vi "Rename InstrumentStudio Plug-In Data File.vi"(0 "configuration":T1, 5 "Plugin Library Path":path, 11 "error in":errorcluster) -> (4 "IS Plugin Data File Path":path, 15 "error out":errorcluster)   [LabVIEW 2021, in "InstrumentStudio Plug-In Editor.lvlib"]
uses:
  InstrumentStudio Plug-In Editor.lvlib
  controls/Data Holder.ctl
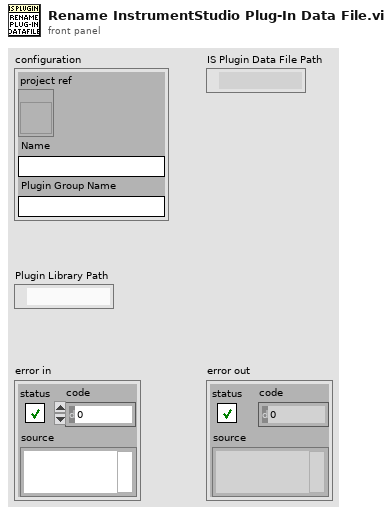
[diagram p1: front panel]
types:
  T1 = typedef "InstrumentStudio Plug-In Editor.lvlib/Data Holder.ctl" = cluster{"project ref":refnum<vi>, "Name":string, "Plugin Group Name":string}
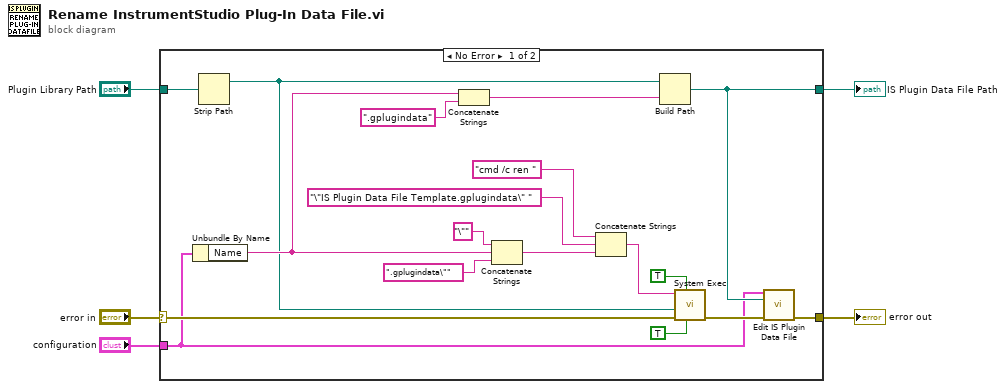
[diagram p0: block diagram]
diagram:
  n1 = case shown="No Error" "error in" {
    selector: "error in" -> [w11 w24]
    tunnel: "Plugin Library Path" -> [w10 _]
    tunnel: [w8 _] -> w3
    tunnel: [w7 w24] -> w2
    tunnel: "configuration" -> [w6 _]
    frame No Error {
      n2 = Unbundle By Name(w6) -> ("Name"=w16:string)
      n3 = Strip Path(path=w10) -> (stripped path=w13:path)  [unwired: 1 out]
      n4 = Concatenate Strings(w16, ".gplugindata" ("string")) -> (w14:string)
      n5 = Concatenate Strings("\"" ("string"), w16, ".gplugindata\"" ("string")) -> (w18:string)
      n6 = Concatenate Strings("cmd /c ren " ("string"), "\"IS Plugin Data File Template.gplugindata\" " ("string"), w18) -> (w21:string)
      n7 = Build Path(base path=w13, name or relative path=w14) -> (appended path=w8:path)
      n8 = call <vilib>:"System Exec.vi"("run minimized? (F)"=TRUE, "wait until completion? (T)"=TRUE, "error in (no error)"=w11, "working directory"=w13, "command line"=w21) -> ("error out"=w9:errorcluster)  [unwired: 3 in, 3 out]
      n9 = call "Edit IS Plugin Data File.vi"("configuration"=w6, "Data File Path"=w8, "error in"=w9) -> ("error out"=w7:errorcluster)  [unwired: 12 in]
    }
    frame Error {
    }
  }
  "error out" <- w2
  "IS Plugin Data File Path" <- w3
